vi "ConvStringFloat (SubVI).vi"(10 "format string":string, 11 "String":string) -> (2 "Numeric":dbl, 3 "output string":string)   [LabVIEW 2017, in "LV_Unicorn.lvlib"]
uses:
  LV_Unicorn.lvlib
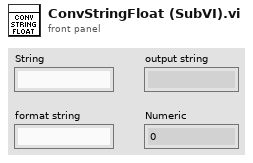
[diagram p1: front panel]
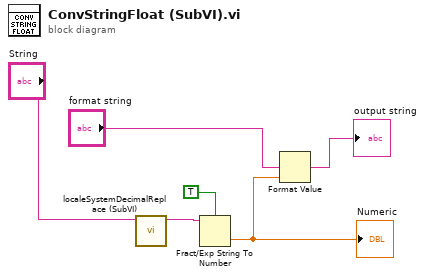
[diagram p0: block diagram]
diagram:
  n1 = call "localeSystemDecimalReplace (SubVI).vi"("String"="String") -> ("result string"=w2:string)  [unwired: 10 in]
  n2 = Fract/Exp String To Number(use system decimal point (T)=TRUE, string=w2) -> (number=w3:dbl)  [unwired: 2 in, 1 out]
  "Numeric" <- w3
  n3 = Format Value(format string="format string", value (0)=w3) -> (output string=→"output string":string)  [unwired: 1 in]
